vi "oax_gsAdd New Events.vi"(1 "event in":string[](array[string])=["initialize"], 2 "new events":string[](array[string])=["initialize"]) -> (0 "event out":string[](array[string])=["initialize"])   [LabVIEW 2017]
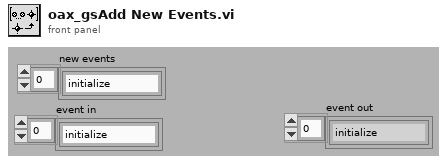
[diagram p1: front panel]
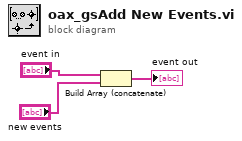
[diagram p0: block diagram]
diagram:
  n1 = Build Array (concatenate)("event in", "new events") -> (→"event out":string[])
